vi "Describe Comparison.vi"(8 "error in (no error)":errorcluster, 9 "Control Value 2":variant, 10 "Control Value 1":variant) -> (0 "error out":errorcluster, 2 "Description":string)   [LabVIEW 2020, in "Identical Inputs Comparator.lvclass"]
uses:
  Identical Inputs Comparator.lvclass
  Core/Comparator/Comparator.lvclass
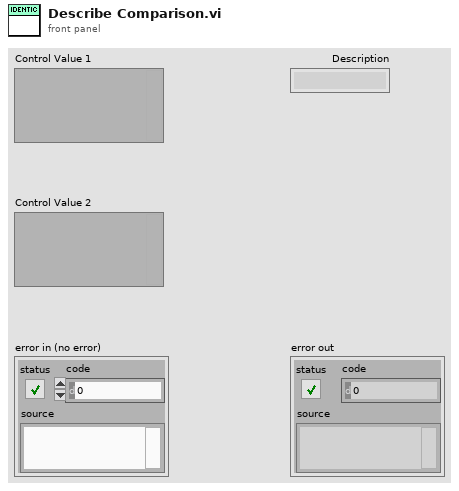
[diagram p1: front panel]
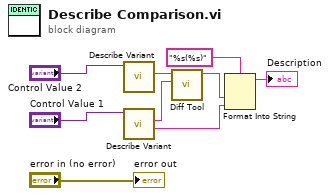
[diagram p0: block diagram]
diagram:
  n1 = call "Describe Variant.vi"("Variant"="Control Value 2") -> ("Description"=w6:string)  [unwired: 8 in, 2 out]
  n2 = call "Describe Variant.vi"("Variant"="Control Value 1") -> ("Type Description"=w1:string, "Description"=w5:string)  [unwired: 8 in, 1 out]
  n3 = call "Diff Tool.vi"("Reference"=w5, "Target"=w6) -> ("Result"=w3:string)  [unwired: 8 in, 1 out]
  n4 = Format Into String(format string="%s(%s)", w3, w1) -> (resulting string=→"Description":string)  [unwired: 2 in, 1 out]
  "error out" <- "error in (no error)"
